vi "Draw.vi"(8 "error in (no error)":errorcluster, 10 "2D Picture in":picture, 11 "Line in":refnum<class "Line.lvclass">) -> (0 "error out":errorcluster, 2 "2D Picture out":picture, 3 "Line out":refnum<class "Line.lvclass">)   [LabVIEW 2021, in "Picture2D.lvlib" / "Line.lvclass"]
uses:
  Line.lvclass
  Line.lvclass/Line.ctl
  Color/Color.lvclass
  Point/Point.lvclass
  Pen/Pen.lvclass
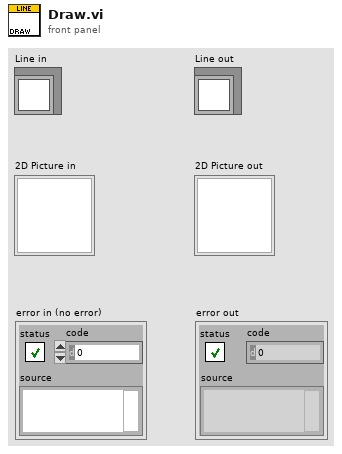
[diagram p1: front panel]
types:
  T1 = cluster{"Width":u16, "Style":enum32{"Solid", "Dash", "Dot", "DashDot", "DashDotDot"}}
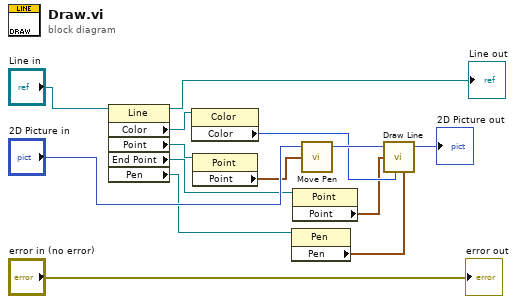
[diagram p0: block diagram]
diagram:
  n1 = property class="Line"(reference="Line in") -> (reference out=→"Line out":refnum<class "Line.lvclass">, "Color"=w7:refnum<class "Color.lvclass">, "Point"=w11:refnum<class "Point.lvclass">, "End Point"=w10:refnum<class "Point.lvclass">, "Pen"=w1:refnum<class "Pen.lvclass">)  [unwired: 1 in, 1 out]
  n2 = property class="Color"(reference=w7) -> ("Color"=w6:u32)  [unwired: 1 in, 2 out]
  n3 = property class="Point"(reference=w11) -> ("Point"=w5:cluster{"x":i16, "y":i16})  [unwired: 1 in, 2 out]
  n4 = property class="Pen"(reference=w1) -> ("Pen"=w4:T1)  [unwired: 1 in, 2 out]
  n5 = property class="Point"(reference=w10) -> ("Point"=w3:cluster{"x":i16, "y":i16})  [unwired: 1 in, 2 out]
  n6 = call <vilib>:"Move Pen.vi"("new position"=w5, "picture"="2D Picture in") -> ("new picture"=w8:picture)  [unwired: 3 in]
  n7 = call <vilib>:"Draw Line.vi"("picture"=w8, "end point"=w3, "color(black)"=w6, "pen"=w4) -> ("new picture"=→"2D Picture out":picture)  [unwired: 5 in]
  "error out" <- "error in (no error)"
